vi "QuadExtraPass (SubVI).vi"(0 "Image":i32[][](array[numeric]), 2 "radial bins/pixel":dbl, 3 "First position":dbl[](array[numeric]), 7 "window":dbl[](array[numeric]), 11 "angularbinlengths":i32[](array[numeric]), 12 "Rcos(phi)[Q]":dbl[][][](array[numeric]), 13 "Rsin(phi)[Q]":dbl[][][](array[numeric]), 14 "# Radial bins":u32) -> (4 "offset measured (pixels)":dbl[](array[numeric]), 6 "radial profile":dbl[](array[numeric]), 10 "New Position (pixels)":dbl[](array[numeric]))   [LabVIEW 2011, in "OfflineTracker.lvlib"]
uses:
  OfflineTracker.lvlib
panel:
  out "Waveform Graph":dbl[](graph)
  out "Position Correction":dbl[](array[numeric])
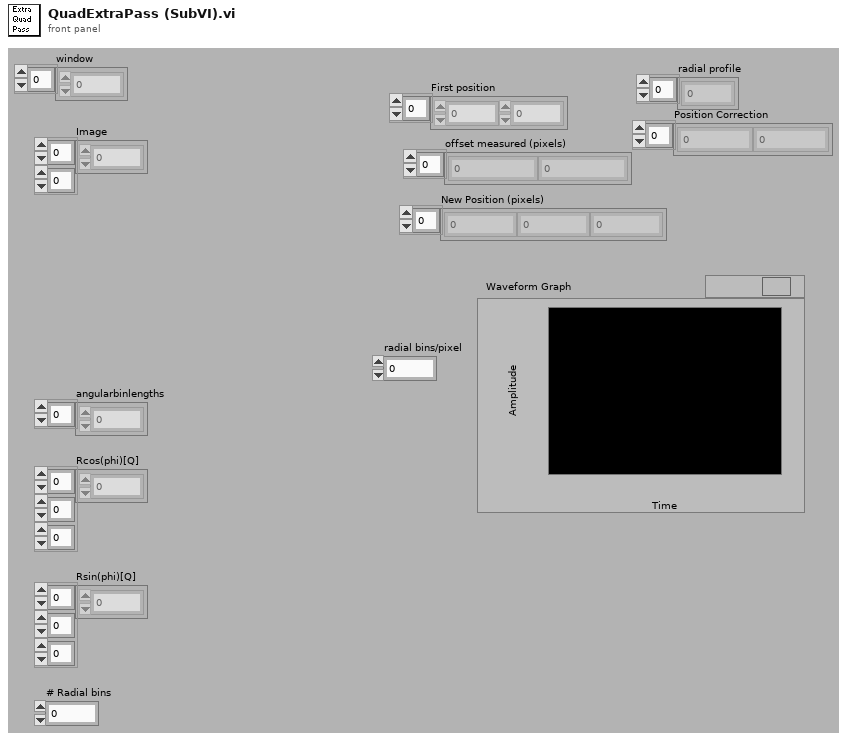
[diagram p1: front panel]
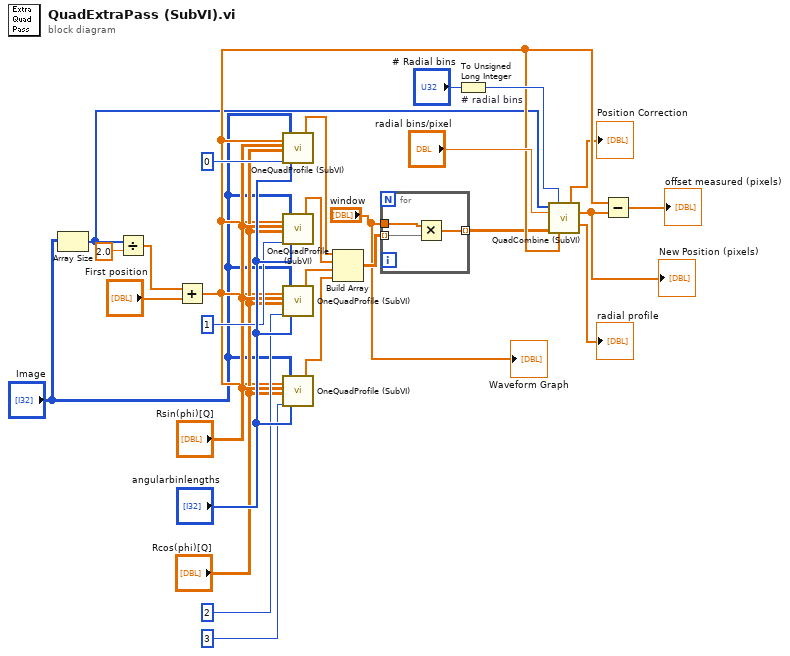
[diagram p0: block diagram]
diagram:
  n1 = Array Size(array="Image") -> (size(s)=w4:i32[])
  n2 = Divide(x=w4, y=2.0 ("median image")) -> (x/y=w7:dbl[])
  n3 = Add(x=w7, y="First position") -> (x+y=w8:dbl[])
  n4 = call "OneQuadProfile (SubVI).vi"("corner-based \ncoordinates (pix)"=w8, "Rsin(phi)[Q]"="Rsin(phi)[Q]", "Rcos(phi)[Q]"="Rcos(phi)[Q]", "Quadrant?"=0 ("Numeric"), "Image"="Image", "lengths"="angularbinlengths") -> ("profile"=w21:dbl[])  [unwired: 4 in, 9 out]
  n5 = call "OneQuadProfile (SubVI).vi"("corner-based \ncoordinates (pix)"=w8, "Rsin(phi)[Q]"="Rsin(phi)[Q]", "Rcos(phi)[Q]"="Rcos(phi)[Q]", "Quadrant?"=1 ("Numeric"), "Image"="Image", "lengths"="angularbinlengths") -> ("profile"=w17:dbl[])  [unwired: 4 in, 9 out]
  n6 = call "OneQuadProfile (SubVI).vi"("corner-based \ncoordinates (pix)"=w8, "Rsin(phi)[Q]"="Rsin(phi)[Q]", "Rcos(phi)[Q]"="Rcos(phi)[Q]", "Quadrant?"=2 ("Numeric"), "Image"="Image", "lengths"="angularbinlengths") -> ("profile"=w20:dbl[])  [unwired: 4 in, 9 out]
  n7 = call "OneQuadProfile (SubVI).vi"("corner-based \ncoordinates (pix)"=w8, "Rsin(phi)[Q]"="Rsin(phi)[Q]", "Rcos(phi)[Q]"="Rcos(phi)[Q]", "Quadrant?"=3 ("Numeric"), "Image"="Image", "lengths"="angularbinlengths") -> ("profile"=w23:dbl[])  [unwired: 4 in, 9 out]
  n8 = Build Array(w21, w17, w20, w23) -> (w22:dbl[][])
  n9 = for {
    tunnel: w22 -> [w30] mode=indexing
    tunnel: [w29] -> w2 mode=indexing
    tunnel: "window" -> [w28]
    n10 = Multiply(x=w28, y=w30) -> (x*y=w29:dbl[])
  }
  n11 = To Unsigned Long Integer "# radial bins"(number="# Radial bins") -> (unsigned 32bit integer=w24:u32)
  n12 = call "QuadCombine (SubVI).vi"("roi"=w4, "# of radial bins"=w24, "radial bins/pixel"="radial bins/pixel", "profiles"=w2, "pre-xy (pixels)"=w8) -> ("Position Correction"=→"Position Correction":dbl[], "Position (pixels)"=w10:dbl[], "radial profile"=→"radial profile":dbl[])  [unwired: 1 in, 7 out]
  "New Position (pixels)" <- w10
  n13 = Subtract(x=w8, y=w10) -> (x-y=→"offset measured (pixels)":dbl[])
  "Waveform Graph" <- "window"
